vi "Import ESI File.vi"(7 "Select a device profile or file path":path, 8 "error in":errorcluster, 9 "Import to RT target":bool, 10 "Import to host PC":bool, 11 "Target IP Address":string) -> (0 "error out":errorcluster, 3 "result out":string[][](array[string]))   [LabVIEW 2019, in "SEECD System Explorer.lvlib"]
uses:
  SEECD System Explorer.lvlib
  <vilib>/nisyscfg/Close (System).vi
  <vilib>/nisyscfg/nisyscfg.lvlib
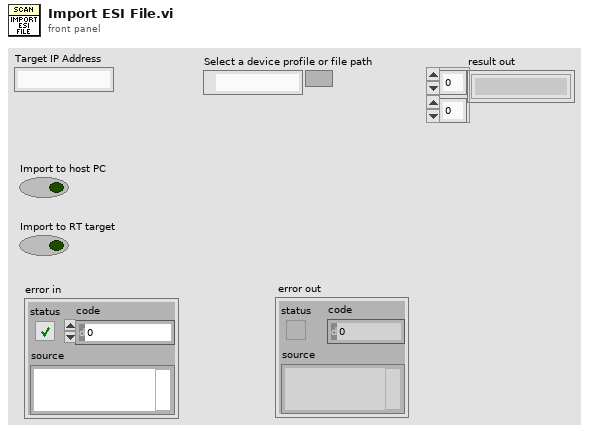
[diagram p1: front panel]
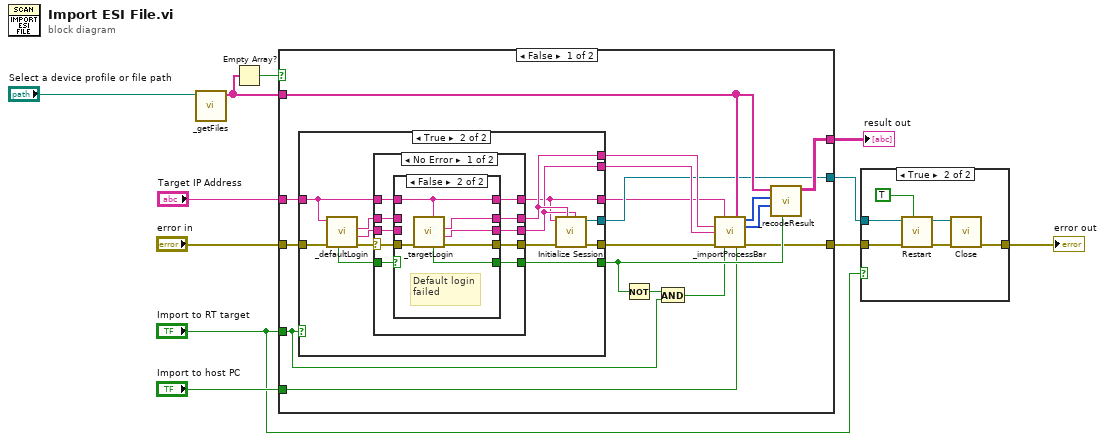
[diagram p0: block diagram]
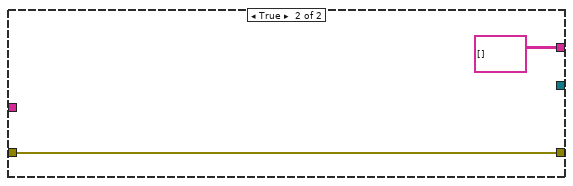
[diagram p6: hidden frame]
diagram:
  n1 = call <resource>:"_getFiles.vi"("Selected path"="Select a device profile or file path") -> ("Import files"=w6:string[])  [unwired: 6 in]
  n2 = Empty Array?(array=w6) -> (empty?=w7:bool)
  n3 = case shown="False" w7 {
    tunnel: [w28 string[][] [] ("result out")] -> w3
    tunnel: w6 -> [w20 _]
    tunnel: "Target IP Address" -> [w21 _]
    tunnel: "error in" -> [w25 w66]
    tunnel: [w16 _] -> w9
    tunnel: "Import to RT target" -> [w14 _]
    tunnel: "Import to host PC" -> [w13 _]
    tunnel: [w15 w66] -> w4
    frame False {
      n4 = case shown="True" w14 {
        tunnel: w21 -> [_ w36]
        tunnel: [_ w32] -> w24
        tunnel: [_ w31] -> w23
        tunnel: [_ w41] -> w27
        tunnel: [_ w33] -> w22
        tunnel: w25 -> [_ w35]
        tunnel: [_ w30] -> w16
        tunnel: [_ w29] -> w12
        frame False {
        }
        frame True {
          n5 = call <resource>:"_defaultLogin.vi"("error in"=w35, "Target IP"=w36) -> ("error out"=w38:errorcluster, "password out"=w39:string, "user name out"=w40:string, "correct login?"=w37:bool)  [unwired: 6 in]
          n6 = case shown="No Error" w38 {
            selector: w38 -> [w45 w65]
            tunnel: [w51 w63] -> w32
            tunnel: [w50 w62] -> w31
            tunnel: [w49 _] -> w41
            tunnel: [w48 w65] -> w34
            tunnel: w40 -> [w47 w63]
            tunnel: w39 -> [w46 w62]
            tunnel: w37 -> [w44 _]
            tunnel: w36 -> [w43 w64]
            tunnel: [w42 w64] -> w29
            frame No Error {
              n7 = case shown="False" w44 {
                tunnel: [w55 w61] -> w51
                tunnel: [w54 w60] -> w50
                tunnel: [w53 w59] -> w48
                tunnel: [_ w58] -> w49
                tunnel: w47 -> [w55 _]
                tunnel: w46 -> [w54 _]
                tunnel: w45 -> [w53 w57]
                tunnel: w43 -> [w52 w56]
                tunnel: [w52 w56] -> w42
                frame True {
                }
                frame False {
                  # "Default login failed"
                  n8 = call <resource>:"_targetLogin.vi"("Target IP"=w56, "error in"=w57) -> ("error out"=w59:errorcluster, "Password out"=w60:string, "Username out"=w61:string, "cancel?"=w58:bool)  [unwired: 6 in]
                }
              }
            }
            frame Error {
            }
          }
          n9 = call <vilib>:"Initialize Session.vi"("Password"=w31, "User Name"=w32, "error in (no error)"=w34, "Target (localhost)"=w29) -> ("error out"=w33:errorcluster, "Session out"=w30:refnum<k21>)  [unwired: 6 in]
        }
      }
      n10 = Not(x=w27) -> (.not. x?=w26:bool)
      n11 = And(x=w26, y=w14) -> (x .and. y?=w17:bool)
      n12 = call "_importProcessBar.vi"("Target IP"=w12, "ProfileSrcPath"=w20, "user name"=w24, "password"=w23, "error in (no error)"=w22, "importTarget?"=w17, "importHost?"=w13) -> ("hostResult"=w19:i32[], "targetResult"=w18:i32[], "error out"=w15:errorcluster)  [unwired: 6 in]
      n13 = call <resource>:"_recodeResult.vi"("cancel?"=w27, "targetResult"=w18, "hostResult"=w19, "Import files"=w20) -> ("result out"=w28:string[][])  [unwired: 7 in]
    }
    frame True {
    }
  }
  "result out" <- w3
  n14 = case shown="True" "Import to RT target" {
    tunnel: w4 -> [w68 w74]
    tunnel: w9 -> [_ w73]
    tunnel: [w68 w69] -> w1
    frame False {
    }
    frame True {
      n15 = call <vilib>:"Restart.vi"("Wait Until Complete (T)"=TRUE, "error in (no error)"=w74, "Session in"=w73) -> ("error out"=w71:errorcluster, "Session out"=w70:refnum<k21>)  [unwired: 6 in, 1 out]
      n16 = call-poly <vilib>:"Close.vi"("error in (no error)"=w71, "Session in"=w70) -> ("error out"=w69:errorcluster)  [unwired: 9 in]
    }
  }
  "error out" <- w1
